vi "Main.vi"() -> ()   [LabVIEW 2021]
uses:
  SQLCLASS/SQLObject.lvclass
panel:
  in  "DataBase":T1={"Value1"=1.0, "Value2"=2.0, "Value3"=3.0, "int"=0, "String"="", "double"=0.0}
  out "Table Control":string[][](table)
  out "error out":errorcluster
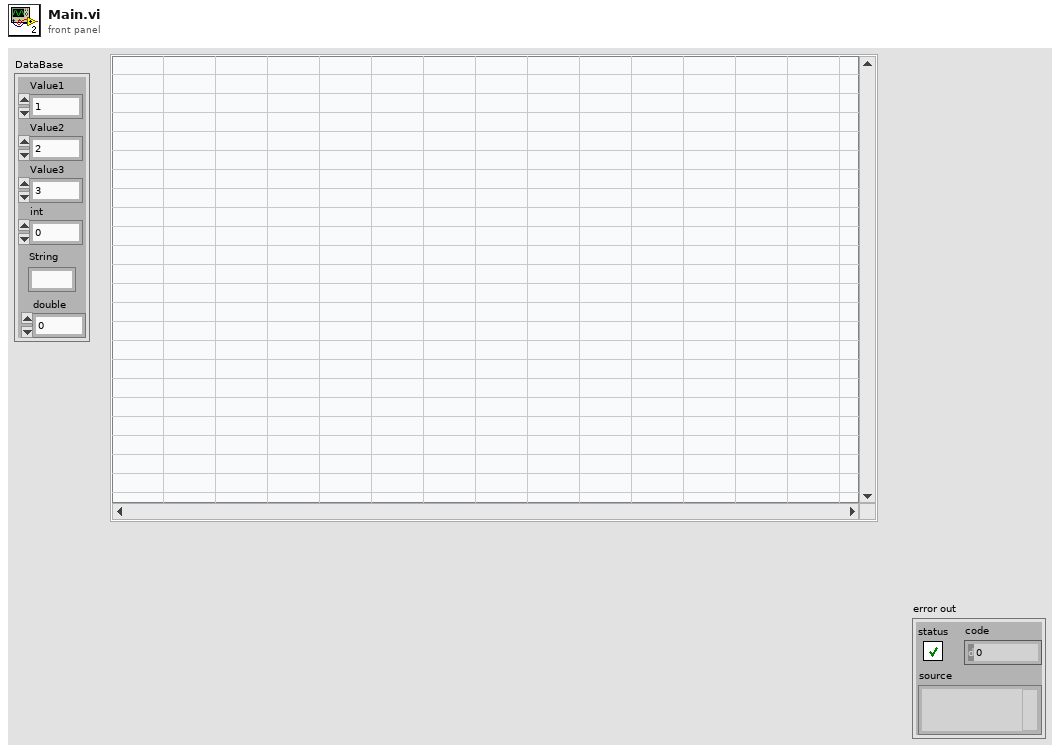
[diagram p1: front panel]
types:
  T1 = cluster{"Value1":dbl, "Value2":dbl, "Value3":dbl, "int":i32, "String":string, "double":dbl}
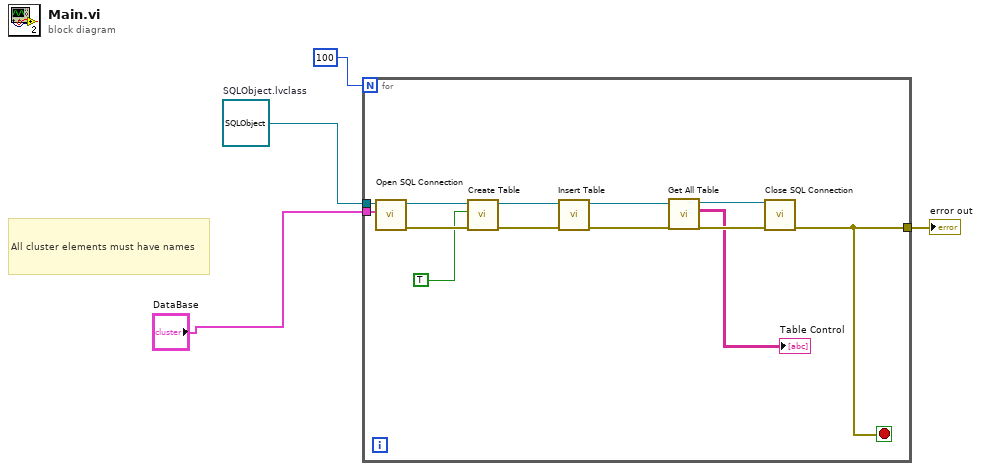
[diagram p0: block diagram]
diagram:
  w4 = refnum<class "SQLObject.lvclass"> refnum  # SQLObject.lvclass
  # "All cluster elements must have names"
  n1 = for {
    N: 100 -> [_]
    tunnel: w4 -> [w12]
    tunnel: "DataBase" -> [w6]
    tunnel: [w5] -> w1
    stop <- w5 stop-if-true
    n2 = call-dynamic "Open SQL Connection.vi"("SQL Data"=w6, "SQLObject in"=w12) -> ("error out"=w9:errorcluster, "SQLObject out"=w11:refnum<class "SQLObject.lvclass">)  [unwired: 7 in, 1 out]
    n3 = call-dynamic "Create Table.vi"("error in (no error)"=w9, "Primary Key?"=TRUE, "SQLObject in"=w11) -> ("error out"=w8:errorcluster, "SQLObject out"=w10:refnum<class "SQLObject.lvclass">)  [unwired: 7 in]
    n4 = call-dynamic "Insert Table.vi"("error in (no error)"=w8, "SQLObject in"=w10) -> ("error out"=w17:errorcluster, "SQLObject out"=w16:refnum<class "SQLObject.lvclass">)  [unwired: 8 in]
    n5 = call-dynamic "Get All Table.vi"("error in (no error)"=w17, "SQLObject in"=w16) -> ("error out"=w14:errorcluster, "Result Set"=→"Table Control":string[][], "SQLObject out"=w15:refnum<class "SQLObject.lvclass">)  [unwired: 7 in]
    n6 = call-dynamic "Close SQL Connection.vi"("error in (no error)"=w14, "SQLObject in"=w15) -> ("error out"=w5:errorcluster)  [unwired: 8 in, 1 out]
  }
  "error out" <- w1
